vi "ex2.vi"() -> ()   [LabVIEW 2022 SP3]
uses:
  <vilib>/Math Plots/2D Math Plots/XY Plot Matrix/XY Plot Matrix Datatype/XY Plot Matrix Datatype.lvclass
  <vilib>/Math Plots/2D Math Plots/2D Feather/2D Feather Datatype/2D Feather Datatype.lvclass
  <vilib>/Math Plots/2D Math Plots/2D Feather/2D Feather Datatype/Public/Plot Helper (Vector).vi
panel:
  in  "Starting Phase":dbl(knob) scale=0.36..360.0
  in  "?":bool
  in  "?":bool
  in  "?":bool
  in  "?":bool
  out "Waveform Graph":dbl[](graph)
  in  "Copy Measurement To Clipboard":bool
  in  "Auto Save The Measurement":bool
  in  "Close After The Measurement":bool
  in  "Enable Auto Scale":bool
  out "Measurement Progress":u8(slide) scale=0.0..100.0
  in  "Status":dbl(knob) scale=0.0..5.0
  # "Status"
  # "Status"
  # "Options"
  # "Starting Phase"
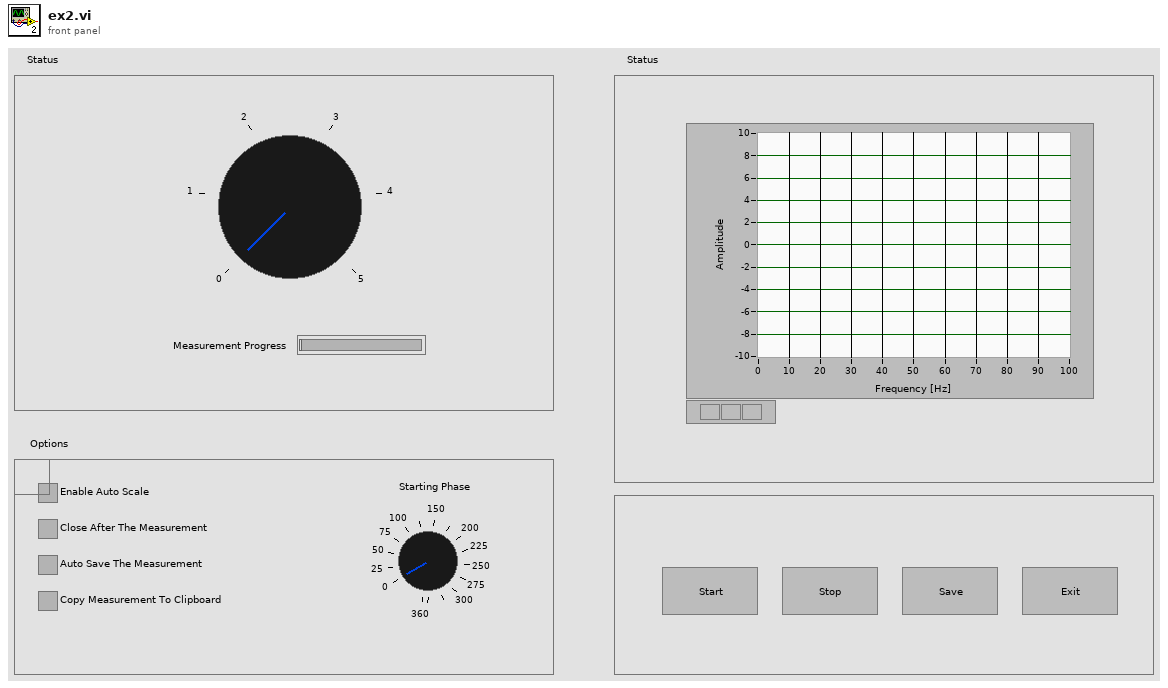
[diagram p1: front panel]
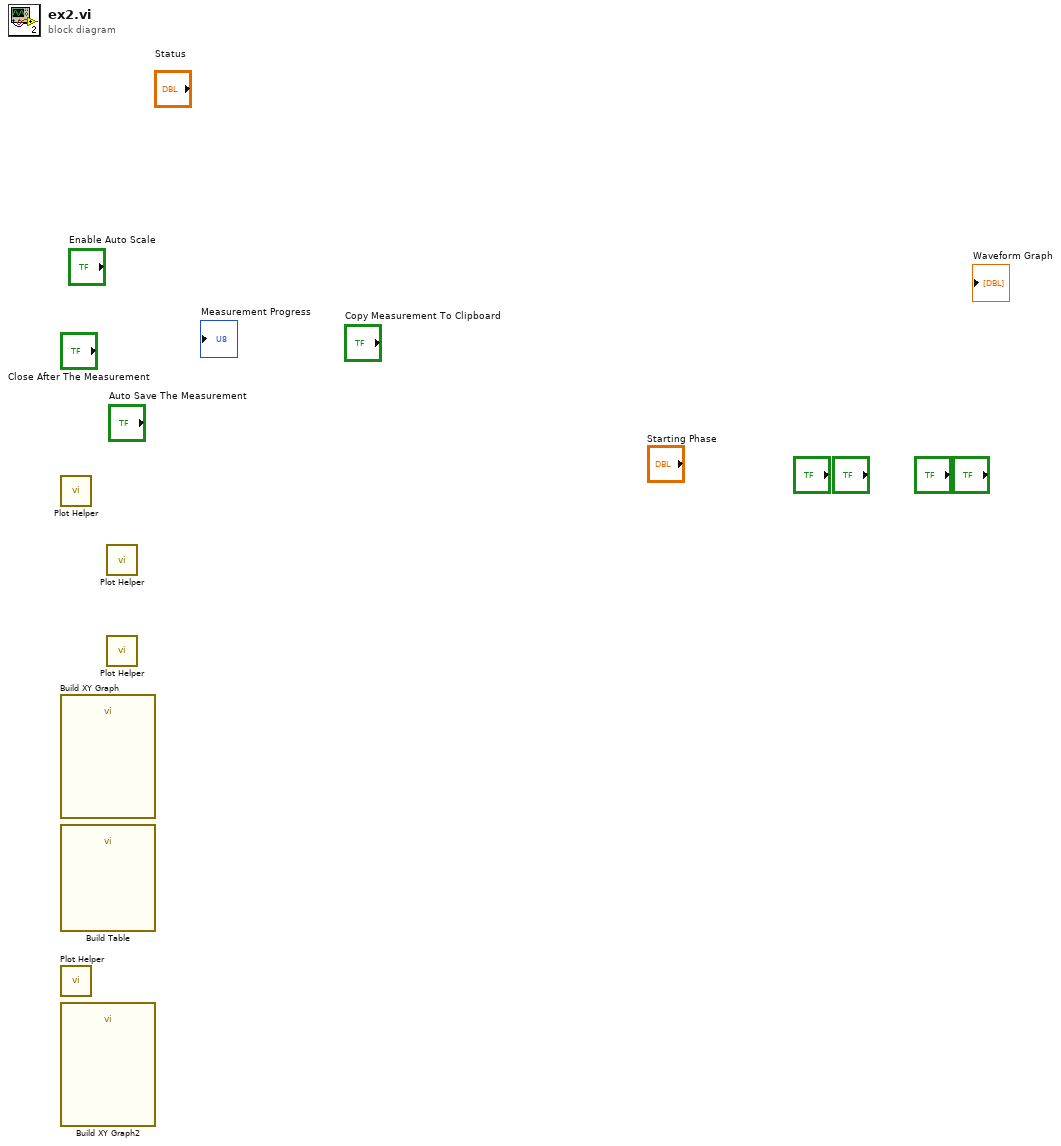
[diagram p0: block diagram]
diagram:
  n1 = call <vilib>:"Plot Helper.vi"() -> ("2D Plotmatrix Class Obj Array out"=w7:refnum<class "XY Plot Matrix Datatype.lvclass">[])  [unwired: 4 in, 7 out]
  n2 = call "Build XY Graph"() -> ("XY Graph"=w4:cluster{"X":dbl[], "Y":dbl[]}[])  [unwired: 10 in, 1 out]
  n3 = call "Build Table"() -> ("Table"=w3:string[][])  [unwired: 5 in, 6 out]
  n4 = call <vilib>:"Plot Helper.vi"() -> ("2D Plotmatrix Class Obj Array out"=w2:refnum<class "XY Plot Matrix Datatype.lvclass">[])  [unwired: 4 in, 7 out]
  n5 = call "Build XY Graph2"() -> ("XY Graph"=w1:cluster{"X":dbl[], "Y":dbl[]}[])  [unwired: 10 in, 1 out]
  n6 = call-poly <vilib>:"Plot Helper.vi"() -> ("2D Plot Class Obj Array out"=w6:refnum<class "2D Plot Datatype.lvclass">[])  [unwired: 4 in, 7 out]
  n7 = call-poly <vilib>:"Plot Helper.vi"() -> ("2D Plot Class Obj Array out"=w5:refnum<class "2D Plot Datatype.lvclass">[])  [unwired: 4 in, 7 out]
